vi "CRC16_2.vi"(11 "buf":u8[](array[numeric]) format="%x") -> (2 "CRCHi":u8 format="%x", 3 "CRCLo":u8 format="%x")   [LabVIEW 2012]
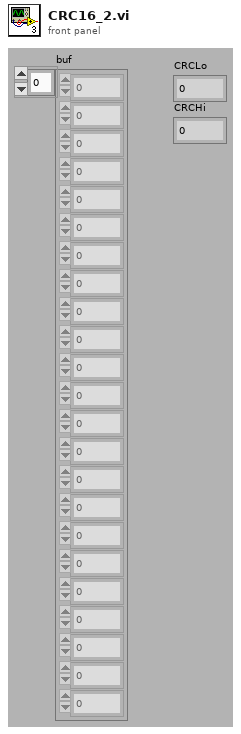
[diagram p1: front panel]
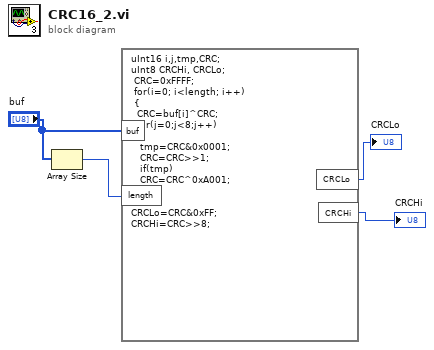
[diagram p0: block diagram]
diagram:
  n1 = Array Size(array="buf") -> (size(s)=w3:i32)
  n2 = formula code="uInt16 i,j,tmp,CRC;\nuInt8 CRCHi, CRCLo;\n\tCRC=0xFFFF;\n\tfor(i=0; i<length; i++)\n\t{\n\t\tCRC=buf[i]^CRC;\n\t\tfor(j=0;j<8;j++)\n\t\t{\t\n\t\t\ttmp=CRC&0x0001;\n\t\t\tCRC=CRC>>1;\n\t\t\tif(tmp)\n\t\t\tCRC=CRC^0xA001;\n\t\t}\n\t}\nCRCLo=CRC&0xFF;\nCRCHi=CRC>>8;"("buf"="buf", "length"=w3) -> ("CRCLo"=→"CRCLo":u8, "CRCHi"=→"CRCHi":u8)
